vi "ClimbExecute2.vi"() -> ()   [LabVIEW 2023]
uses:
  <vilib>/Rock Robotics/WPI/ThirdParty/JAS_Junk/TrajLib/MathUtil_Clamp.vi
  <vilib>/Rock Robotics/WPI/ThirdParty/JAS_Junk/TrajLib/VI/numCmd_ObtainQueue_OneDbl.vi
  <vilib>/Rock Robotics/Network Tables/NT Write Number.vi
  <vilib>/Rock Robotics/Network Tables/NT Write Boolean.vi
  <vilib>/Rock Robotics/WPI/ThirdParty/JAS_Junk/TrajLib/Trajectory_Library.lvlib
panel:
  in  "Ready1":bool=TRUE
  out "Do Command 1":bool
  out "Do Command 2":bool
  out "Do Cancel":bool
  in  "Ready2":bool=TRUE
  in  "Ready3":bool=TRUE
  in  "Ready4":bool=TRUE
  in  "Ready5":bool=TRUE
  in  "Ready6":bool=TRUE
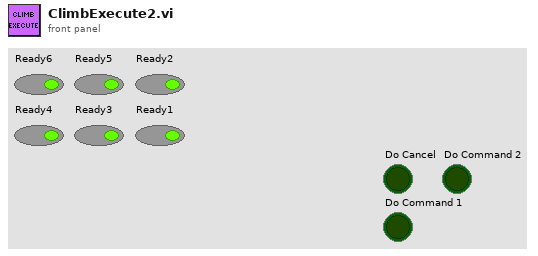
[diagram p1: front panel]
types:
  T1 = typedef "WPI_MotorControlDeviceRef.ctl" = cluster{"DeviceStatus":errorcluster, "Type":T2, "PWM":cluster{"PWM Channel":T3, "DeadBand":T4}, "CAN":cluster{"Device Number":u8, "SetOutput VI Ref":variant, "GetOutput VI Ref":variant, "Enable VI Ref":variant, "Disable VI Ref":variant, "Data":variant}, "Invert":bool, "DIO PWM":cluster{"PWM \"Enable\" Channel":T3, "DIOChannel":T5, "PWM Rate":dbl}}
  T2 = typedef "WPI_MotorControlType.ctl" = enum16{"PWM", "CAN", "DIO PWM"}
  T3 = typedef "FPGA_DIOPWMChannel.ctl" = enum8{"PWM 0", "PWM 1", "PWM 2", "PWM 3", "PWM 4", "PWM 5", "PWM 6", "PWM 7", "PWM 8", "PWM 9", "PWM MXP 0", "PWM MXP 1", "PWM MXP 2", "PWM MXP 3", "PWM MXP 4", "PWM MXP 5", "PWM MXP 6", "PWM MXP 7", "PWM MXP 8", "PWM MXP 9", "Invalid"}
  T4 = typedef "WPI_PWMDeadband.ctl" = cluster{"Name":string, "maxPositivePwm":i32, "minPositivePwm":i32, "centerPwm":i32, "maxNegativePwm":i32, "minNegativePwm":i32, "angularRange":u16}
  T5 = typedef "FPGA_DIOChannel.ctl" = enum8{"DIO 0", "DIO 1", "DIO 2", "DIO 3", "DIO 4", "DIO 5", "DIO 6", "DIO 7", "DIO 8", "DIO 9", "DIO MXP 0", "DIO MXP 1", "DIO MXP 2", "DIO MXP 3", "DIO MXP 4", "DIO MXP 5", "DIO MXP 6", "DIO MXP 7", "DIO MXP 8", "DIO MXP 9", "DIO MXP 10", "DIO MXP 11", "DIO MXP 12", "DIO MXP 13", "DIO MXP 14", "DIO MXP 15", "SPI Port CS1", "SPI Port CS2", "SPI Port CS3", "SPI Port MISO", "SPI Port MOSI", "Invalid"}
  T6 = typedef "Trajectory_Library.lvlib/PosCtrl_Tuning_Type.ctl" = cluster{"Slope":dbl, "Offset":dbl, "Error Deadband":dbl, "At Reference Count":i32, "Negate Output":bool, "Max Allowd Position":dbl, "Min Allowd Position":dbl}
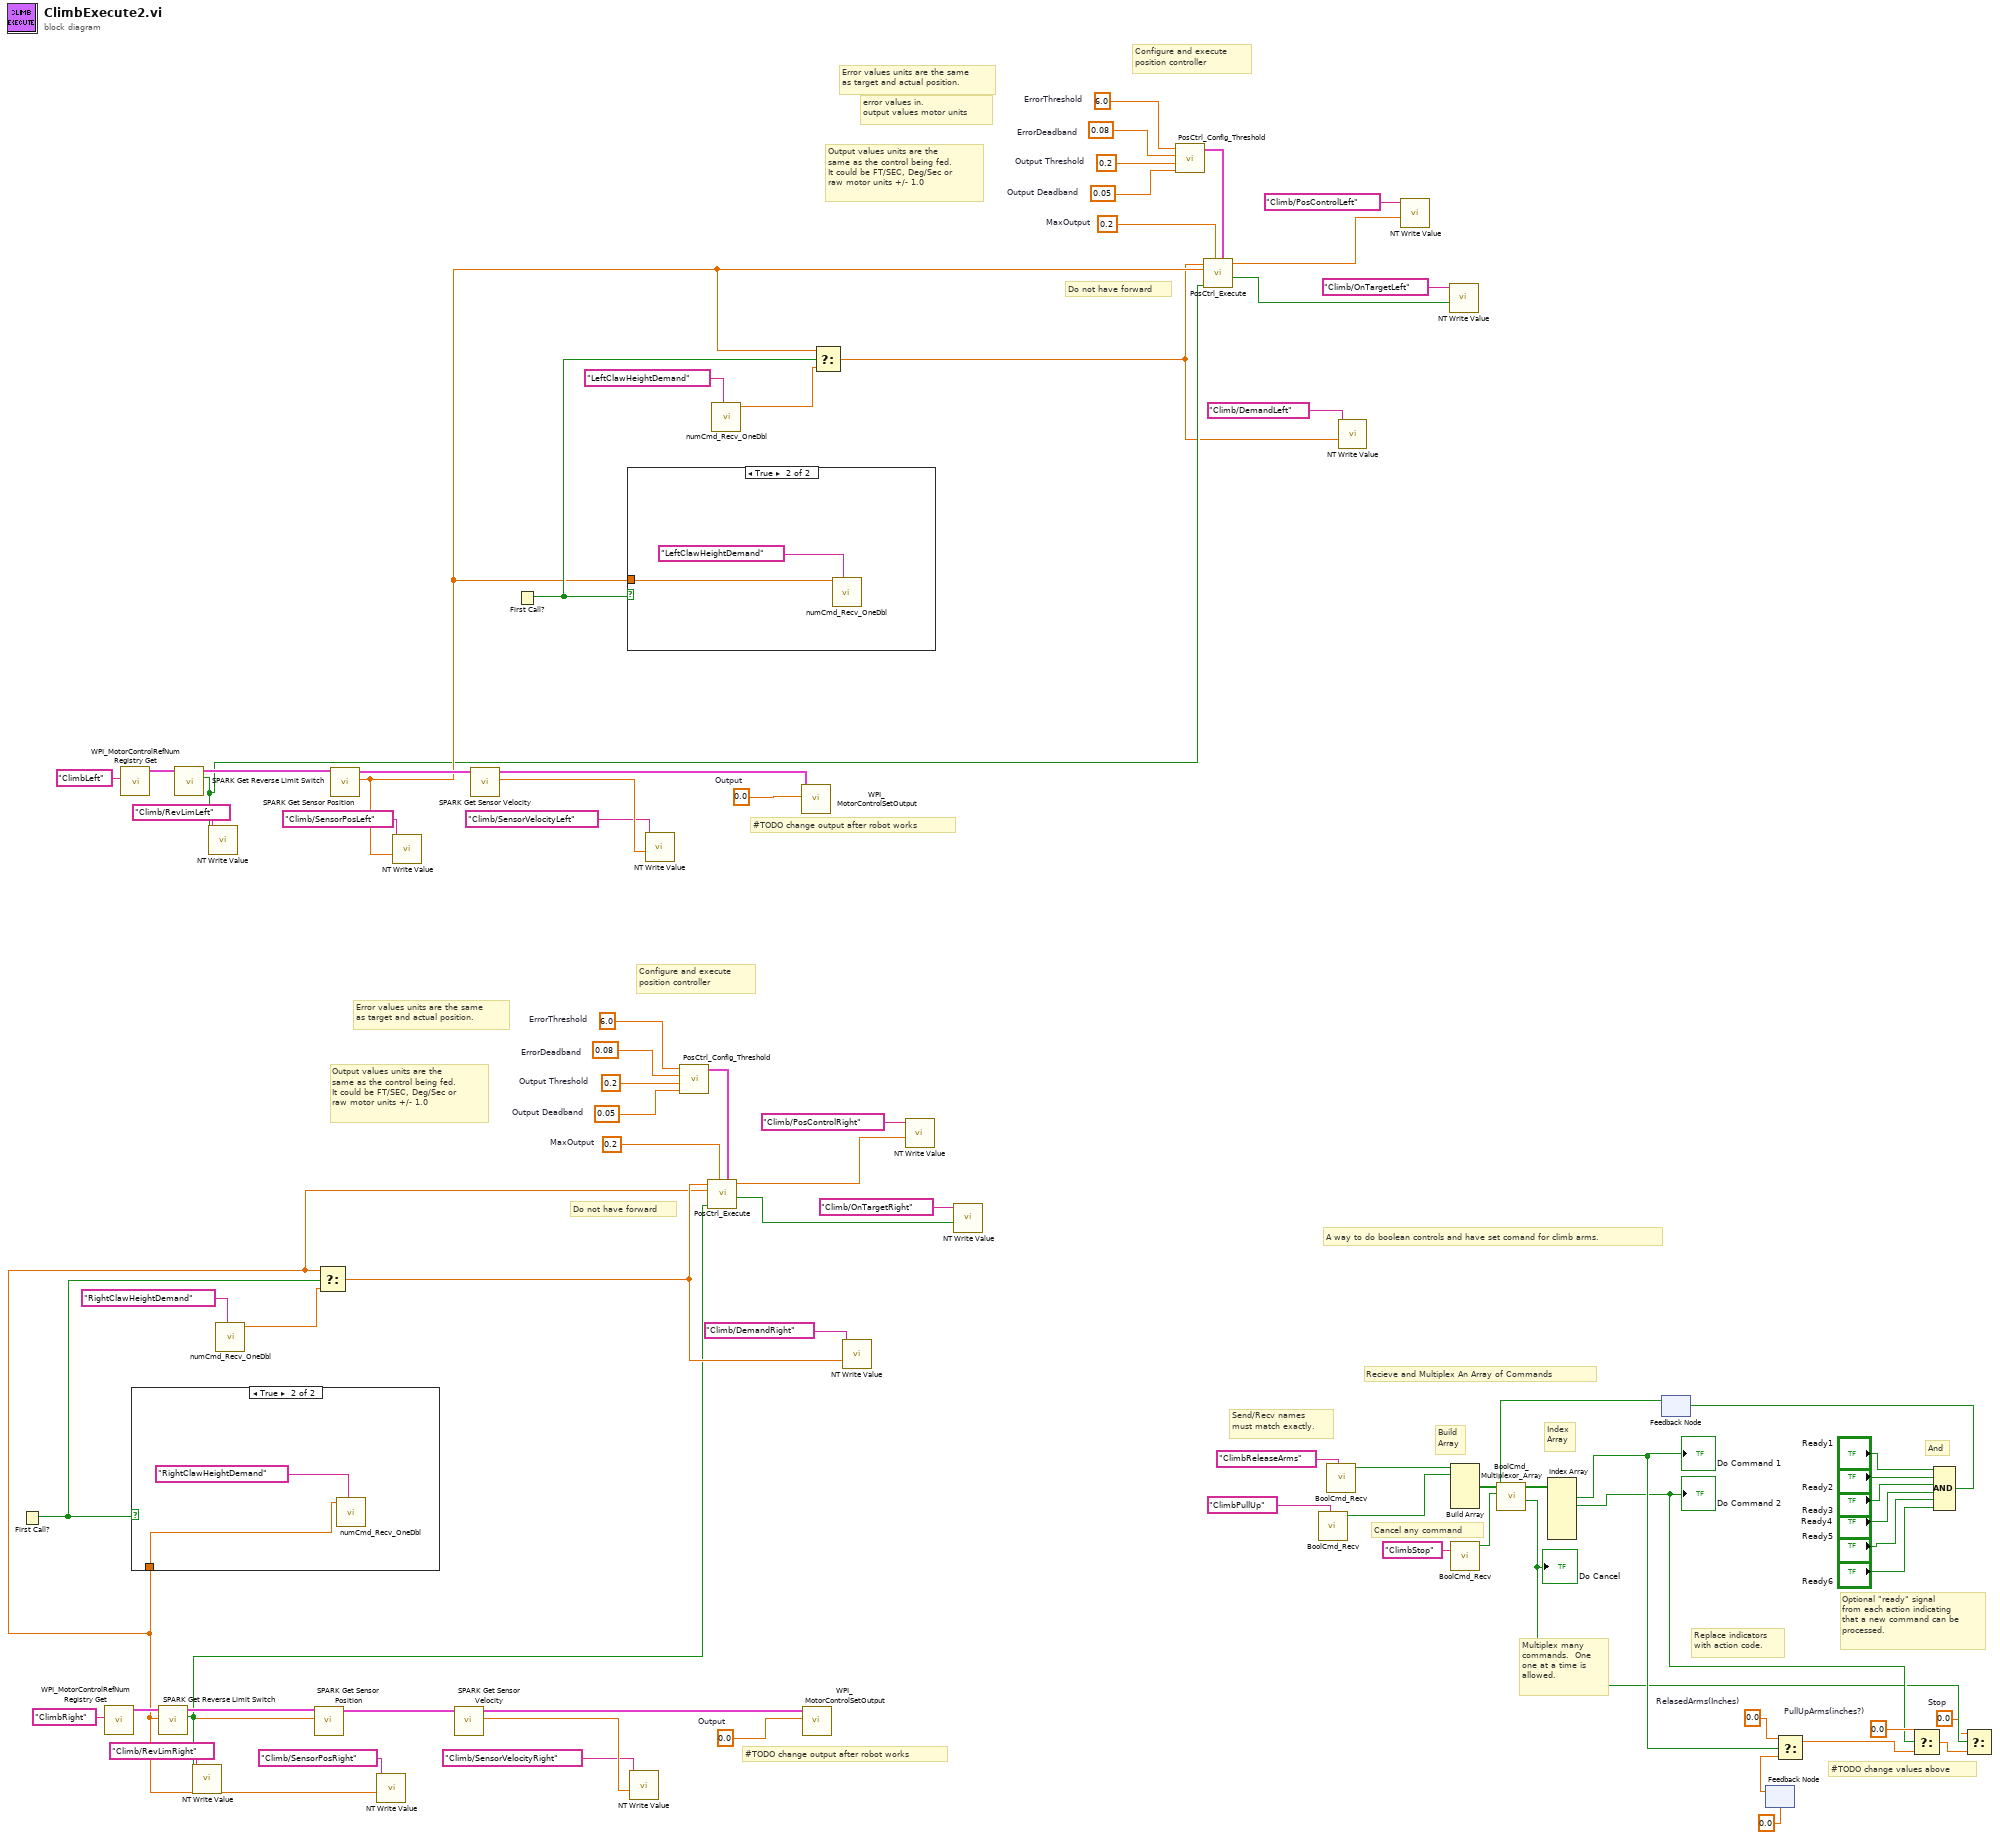
[diagram p0: block diagram]
diagram:
  w5 = 0.0  # Stop
  w8 = 0.0  # PullUpArms(inches?)
  w9 = 0.0  # RelasedArms(Inches)
  w28 = 0.0  # Output
  w45 = 0.2  # MaxOutput
  w43 = 6.0  # ErrorThreshold
  w42 = 0.08  # ErrorDeadband
  w41 = 0.2  # Output Threshold
  w40 = 0.05  # Output Deadband
  w52 = 0.0  # Output
  w80 = 0.2  # MaxOutput
  w78 = 6.0  # ErrorThreshold
  w77 = 0.08  # ErrorDeadband
  w76 = 0.2  # Output Threshold
  w75 = 0.05  # Output Deadband
  # "A way to do boolean controls and have set comand for climb arms."
  # "#TODO change values above"
  # "And"
  # "Cancel any command"
  # "Index\nArray"
  # "Build\nArray"
  # "Replace indicators\nwith action code."
  # "Optional \"ready\" signal\nfrom each action indicating\nthat a new command can be\nprocessed."
  # "Multiplex many\ncommands.  One\none at a time is \nallowed."
  # "Send/Recv names\nmust match exactly."
  # "Recieve and Multiplex An Array of Commands"
  # "error values in.\noutput values motor units"
  # "#TODO change output after robot works"
  # "Do not have forward"
  # "Output values units are the\nsame as the control being fed.  \nIt could be FT/SEC, Deg/Sec or\nraw motor units +/- 1.0"
  # "Error values units are the same \nas target and actual position."
  # "Configure and execute \nposition controller"
  # "#TODO change output after robot works"
  # "Do not have forward"
  # "Output values units are the\nsame as the control being fed.  \nIt could be FT/SEC, Deg/Sec or\nraw motor units +/- 1.0"
  # "Error values units are the same \nas target and actual position."
  # "Configure and execute \nposition controller"
  n1 = First Call?() -> (First Call?: T/F=w39:bool)
  n2 = call <vilib>:"WPI_MotorControlRefNum Registry Get.vi"("refnum name"="ClimbRight") -> ("MotorControlDevRef"=w66:T1)  [unwired: 9 in, 1 out]
  n3 = call <vilib>:"WPI_MotorControlRefNum Registry Get.vi"("refnum name"="ClimbLeft") -> ("MotorControlDevRef"=w74:T1)  [unwired: 9 in, 1 out]
  n4 = call <vilib>:"SPARK Get Reverse Limit Switch.vi"("MotorControlDevRef in"=w66) -> ("Hard Limit Rev"=w31:bool, "MotorControlDevRef out"=w63:T1)  [unwired: 7 in, 2 out]
  n5 = call <vilib>:"SPARK Get Reverse Limit Switch.vi"("MotorControlDevRef in"=w74) -> ("Hard Limit Rev"=w54:bool, "MotorControlDevRef out"=w71:T1)  [unwired: 7 in, 2 out]
  n6 = call-poly <vilib>:"NT Write Value.vi"("value"=w31, "name"="Climb/RevLimRight") -> ()  [unwired: 9 in, 1 out]
  n7 = call-poly <vilib>:"NT Write Value.vi"("value"=w54, "name"="Climb/RevLimLeft") -> ()  [unwired: 9 in, 1 out]
  n8 = call <vilib>:"numCmd_Recv_OneDbl.vi"("Command Name"="RightClawHeightDemand") -> ("Value"=w37:dbl)  [unwired: 8 in, 2 out]
  n9 = call <vilib>:"SPARK Get Sensor Position.vi"("MotorControlDevRef in"=w63) -> ("Sensor Position"=w30:dbl, "MotorControlDevRef out"=w65:T1)  [unwired: 7 in, 2 out]
  n10 = case shown="True" w39 {
    tunnel: w30 -> [_ w81]
    frame False {
    }
    frame True {
      n11 = call <vilib>:"numCmd_Recv_OneDbl.vi"("Command Name"="RightClawHeightDemand", "Initial Value"=w81) -> ()  [unwired: 7 in, 3 out]
    }
  }
  n12 = Select(t=w30, s=w39, f=w37) -> (s? t:f=w36:dbl)
  n13 = call <vilib>:"SPARK Get Sensor Position.vi"("MotorControlDevRef in"=w71) -> ("Sensor Position"=w57:dbl, "MotorControlDevRef out"=w73:T1)  [unwired: 7 in, 2 out]
  n14 = call-poly <vilib>:"NT Write Value.vi"("value"=w30, "name"="Climb/SensorPosRight") -> ()  [unwired: 9 in, 1 out]
  n15 = call-poly <vilib>:"NT Write Value.vi"("value"=w57, "name"="Climb/SensorPosLeft") -> ()  [unwired: 9 in, 1 out]
  n16 = call <vilib>:"SPARK Get Sensor Velocity.vi"("MotorControlDevRef in"=w65) -> ("Sensor Velocity"=w60:dbl, "MotorControlDevRef out"=w27:T1)  [unwired: 7 in, 2 out]
  n17 = call <vilib>:"SPARK Get Sensor Velocity.vi"("MotorControlDevRef in"=w73) -> ("Sensor Velocity"=w68:dbl, "MotorControlDevRef out"=w53:T1)  [unwired: 7 in, 2 out]
  n18 = First Call?() -> (First Call?: T/F=w58:bool)
  n19 = case shown="True" w58 {
    tunnel: w57 -> [_ w83]
    frame False {
    }
    frame True {
      n20 = call <vilib>:"numCmd_Recv_OneDbl.vi"("Command Name"="LeftClawHeightDemand", "Initial Value"=w83) -> ()  [unwired: 7 in, 3 out]
    }
  }
  n21 = call-poly <vilib>:"NT Write Value.vi"("value"=w60, "name"="Climb/SensorVelocityRight") -> ()  [unwired: 9 in, 1 out]
  n22 = call-poly <vilib>:"NT Write Value.vi"("value"=w68, "name"="Climb/SensorVelocityLeft") -> ()  [unwired: 9 in, 1 out]
  n23 = call <vilib>:"PosCtrl_Config_Threshold.vi"("Output Deadband"=w40, "Output Threshold"=w41, "ErrorDeadband"=w42, "ErrorThreshold"=w43) -> ("PosCtrl_Config_Params"=w44:T6)  [unwired: 7 in]
  n24 = call <vilib>:"PosCtrl_Execute.vi"("PosCtrl_Config_Params"=w44, "MaxOutput"=w45, "Rev Limit Switch"=w31, "CurrentPosition"=w30, "TargetPosition"=w36) -> ("OnTarget"=w33:bool, "Output"=w34:dbl)  [unwired: 4 in, 1 out]
  n25 = call <vilib>:"numCmd_Recv_OneDbl.vi"("Command Name"="LeftClawHeightDemand") -> ("Value"=w55:dbl)  [unwired: 8 in, 2 out]
  n26 = call <vilib>:"WPI_MotorControlSetOutput.vi"("Output"=w52, "MotorControlDevRef"=w53) -> ()  [unwired: 7 in, 3 out]
  n27 = call <vilib>:"WPI_MotorControlSetOutput.vi"("Output"=w28, "MotorControlDevRef"=w27) -> ()  [unwired: 7 in, 3 out]
  n28 = Select(t=w57, s=w58, f=w55) -> (s? t:f=w51:dbl)
  n29 = call-poly <vilib>:"NT Write Value.vi"("value"=w36, "name"="Climb/DemandRight") -> ()  [unwired: 9 in, 1 out]
  n30 = call-poly <vilib>:"NT Write Value.vi"("value"=w34, "name"="Climb/PosControlRight") -> ()  [unwired: 9 in, 1 out]
  n31 = call-poly <vilib>:"NT Write Value.vi"("value"=w33, "name"="Climb/OnTargetRight") -> ()  [unwired: 9 in, 1 out]
  n32 = call <vilib>:"PosCtrl_Config_Threshold.vi"("Output Deadband"=w75, "Output Threshold"=w76, "ErrorDeadband"=w77, "ErrorThreshold"=w78) -> ("PosCtrl_Config_Params"=w79:T6)  [unwired: 7 in]
  n33 = call <vilib>:"PosCtrl_Execute.vi"("PosCtrl_Config_Params"=w79, "MaxOutput"=w80, "Rev Limit Switch"=w54, "CurrentPosition"=w57, "TargetPosition"=w51) -> ("OnTarget"=w47:bool, "Output"=w49:dbl)  [unwired: 4 in, 1 out]
  n34 = call <vilib>:"BoolCmd_Recv.vi"("Command Name"="ClimbPullUp") -> ("New Request"=w3:bool)  [unwired: 9 in, 1 out]
  n35 = call <vilib>:"BoolCmd_Recv.vi"("Command Name"="ClimbReleaseArms") -> ("New Request"=w21:bool)  [unwired: 9 in, 1 out]
  n36 = call-poly <vilib>:"NT Write Value.vi"("value"=w51, "name"="Climb/DemandLeft") -> ()  [unwired: 9 in, 1 out]
  n37 = call-poly <vilib>:"NT Write Value.vi"("value"=w49, "name"="Climb/PosControlLeft") -> ()  [unwired: 9 in, 1 out]
  n38 = call-poly <vilib>:"NT Write Value.vi"("value"=w47, "name"="Climb/OnTargetLeft") -> ()  [unwired: 9 in, 1 out]
  n39 = Build Array(w21, w3) -> (w20:bool[])  [unwired: 4 in]
  n40 = call <vilib>:"BoolCmd_Recv.vi"("Command Name"="ClimbStop") -> ("New Request"=w15:bool)  [unwired: 9 in, 1 out]
  n41 = feedback #1() -> (w19:bool)  [unwired: 1 in]
  n42 = call <vilib>:"BoolCmd_Multiplexor_Array.vi"("Ready"=w19, "Command Cancel"=w15, "Commands"=w20) -> ("Do Cancel"=w6:bool, "Do Command"=w22:bool[])  [unwired: 7 in]
  "Do Cancel" <- w6
  n43 = Index Array(array=w22) -> (element #1=w12:bool, element #2=w7:bool)  [unwired: 6 in, 4 out]
  "Do Command 1" <- w12
  "Do Command 2" <- w7
  n44 = feedback-in #2() -> ()  [unwired: 1 out]
  n45 = feedback #2(0.0 ("false")) -> (w1:dbl)
  n46 = Select(t=w9, s=w12, f=w1) -> (s? t:f=w11:dbl)
  n47 = Select(t=w8, s=w7, f=w11) -> (s? t:f=w10:dbl)
  n48 = Compound Arithmetic op=AND("Ready1", "Ready2", "Ready3", "Ready4", "Ready5", "Ready6") -> (w18:bool)
  n49 = feedback-in #1(w18) -> ()
  n50 = Select(t=w5, s=w6, f=w10) -> ()  [unwired: 1 out]
